vi "Send Pulse.vi"(8 "error in (no error)":errorcluster, 11 "SPARC4_GUI in":refnum<class "SPARC4_GUI.lvclass">) -> (0 "error out":errorcluster, 3 "SPARC4_GUI out":refnum<class "SPARC4_GUI.lvclass">)   [LabVIEW 2018, in "SPARC4_GUI.lvclass"]
uses:
  SPARC4_GUI.lvclass
  SPARC4_GUI.lvclass/SPARC4_GUI.ctl
  Channel GUI/Channel GUI.lvclass/Channel GUI.ctl
  State Machine/State Machine.lvclass
  Sync Box/Sync Box.lvclass
  Channel GUI/Channel GUI.lvclass
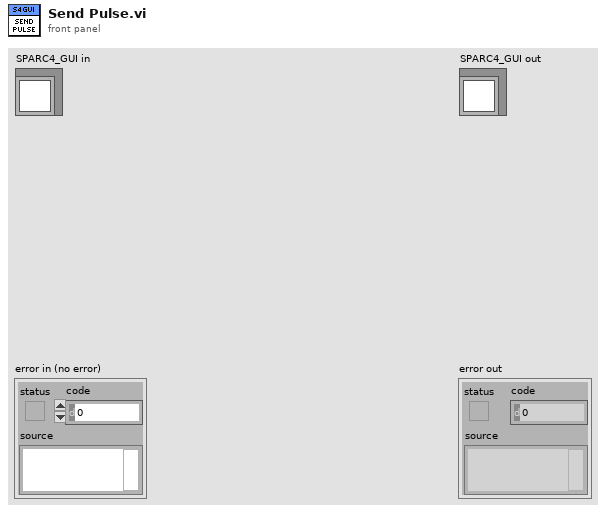
[diagram p1: front panel]
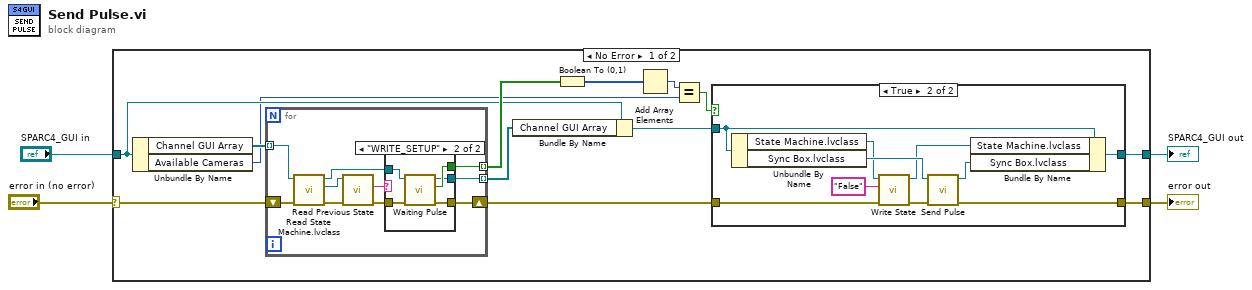
[diagram p0: block diagram]
diagram:
  n1 = case shown="No Error" "error in (no error)" {
    selector: "error in (no error)" -> [w16 w48]
    tunnel: [w11 w48] -> w3
    tunnel: [w10 w47] -> w1
    tunnel: "SPARC4_GUI in" -> [w8 w47]
    frame No Error {
      n2 = Unbundle By Name(w8) -> ("Channel GUI Array"=w17:refnum<class "Channel GUI.lvclass">[], "Available Cameras"=w5:u8)
      n3 = for {
        tunnel: w17 -> [w39] mode=indexing
        tunnel: [w31] -> w15 mode=indexing
        shift-right: [w32] -> w6
        shift-left: w16 -> [w38]
        tunnel: [w30] -> w9 mode=indexing
        n4 = call "Read State Machine.lvclass.vi"("error in (no error)"=w38, "Channel GUI in"=w39) -> ("error out"=w37:errorcluster, "State Machine.lvclass"=w36:refnum<class "State Machine.lvclass">, "Channel GUI out"=w33:refnum<class "Channel GUI.lvclass">)  [unwired: 7 in]
        n5 = call-dynamic "Read Previous State.vi"("error in (no error)"=w37, "State Machine in"=w36) -> ("error out"=w34:errorcluster, "Previous State"=w35:string)  [unwired: 7 in, 1 out]
        n6 = case shown="\"WRITE_SETUP\"" w35 {
          tunnel: w34 -> [w41 w46]
          tunnel: w33 -> [w40 w45]
          tunnel: [w41 w44] -> w32
          tunnel: [_ w43] -> w31
          tunnel: [w40 w42] -> w30
          frame "False", Default {
          }
          frame "WRITE_SETUP" {
            n7 = call "Waiting Pulse.vi"("error in (no error)"=w46, "Channel GUI in"=w45) -> ("error out"=w44:errorcluster, "waiting pulse ?"=w43:bool, "Channel GUI out"=w42:refnum<class "Channel GUI.lvclass">)  [unwired: 7 in]
          }
        }
      }
      n8 = Bundle By Name(cluster=w8, "Channel GUI Array"=w9) -> (w7:refnum<class "SPARC4_GUI.lvclass">)
      n9 = Boolean To (0,1)(Boolean=w15) -> (0, 1=w14:i16[])
      n10 = Add Array Elements(numeric array=w14) -> (sum=w13:i16)
      n11 = Equal?(x=w13, y=w5) -> (x = y?=w12:bool)
      n12 = case shown="True" w12 {
        tunnel: w6 -> [w19 w24]
        tunnel: [w19 w29] -> w11
        tunnel: w7 -> [w18 w26]
        tunnel: [w18 w25] -> w10
        frame False {
        }
        frame True {
          n13 = Unbundle By Name(w26) -> ("State Machine.lvclass"=w21:refnum<class "State Machine.lvclass">, "Sync Box.lvclass"=w28:refnum<class "Sync Box.lvclass">)
          n14 = call-dynamic "Write State.vi"("error in (no error)"=w24, "State"="False", "State Machine in"=w21) -> ("error out"=w23:errorcluster, "State Machine out"=w22:refnum<class "State Machine.lvclass">)  [unwired: 7 in]
          n15 = call "Send Pulse.vi"("error in (no error)"=w23, "Sync Box in"=w28) -> ("error out"=w29:errorcluster, "Sync Box out"=w27:refnum<class "Sync Box.lvclass">)  [unwired: 8 in]
          n16 = Bundle By Name(cluster=w26, "State Machine.lvclass"=w22, "Sync Box.lvclass"=w27) -> (w25:refnum<class "SPARC4_GUI.lvclass">)
        }
      }
    }
    frame Error {
    }
  }
  "error out" <- w3
  "SPARC4_GUI out" <- w1
